vi "Write baud rate (9600).vi"(8 "error in (no error)":errorcluster, 10 "baud rate (9600)":u32=38400, 11 "T560Session in":refnum<class "T560Session.lvclass">) -> (0 "error out":errorcluster, 3 "T560Session out":refnum<class "T560Session.lvclass">)   [LabVIEW 2020, in "T560Session.lvclass"]
uses:
  T560Session.lvclass
  T560Session.lvclass/T560Session.ctl
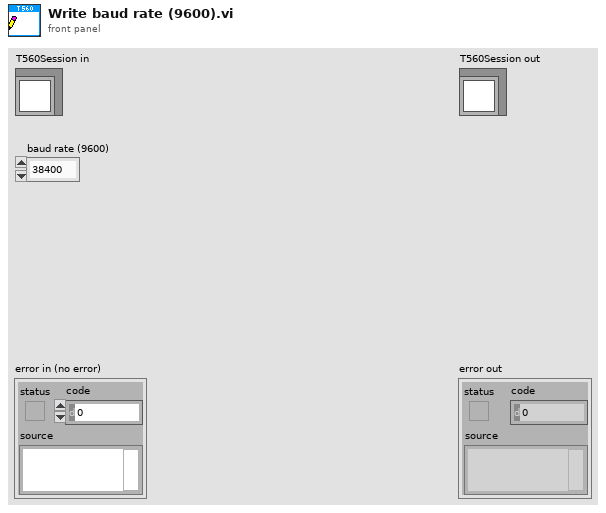
[diagram p1: front panel]
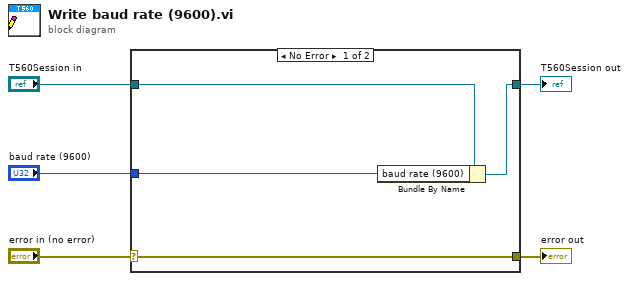
[diagram p0: block diagram]
diagram:
  n1 = case shown="No Error" "error in (no error)" {
    selector: "error in (no error)" -> [w9 w10]
    tunnel: [w9 w10] -> w4
    tunnel: [w7 w11] -> w2
    tunnel: "T560Session in" -> [w8 w11]
    tunnel: "baud rate (9600)" -> [w6 _]
    frame No Error {
      n2 = Bundle By Name(cluster=w8, "baud rate (9600)"=w6) -> (w7:refnum<class "T560Session.lvclass">)
    }
    frame Error {
    }
  }
  "error out" <- w4
  "T560Session out" <- w2
